vi "Lock Subpanel.vi"(8 "error in (no error)":errorcluster, 11 "Subpanel in":refnum<class "Subpanel.lvclass">) -> (0 "error out":errorcluster, 2 "semaphore":T1)   [LabVIEW 2017, in "MGI-Panel Manager.lvlib" / "Subpanel.lvclass"]
uses:
  Subpanel.lvclass
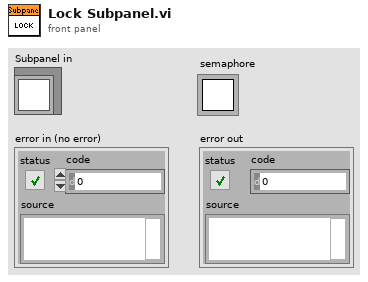
[diagram p1: front panel]
types:
  T1 = typedef "Semaphore RefNum" = refnum<k1>
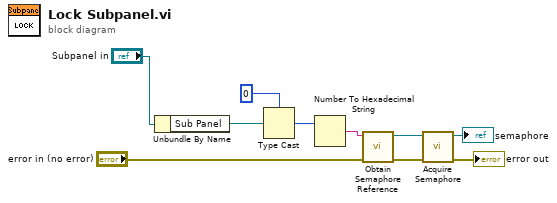
[diagram p0: block diagram]
diagram:
  n1 = Unbundle By Name("Subpanel in") -> ("Sub Panel"=w8:refnum<vi>)
  n2 = Type Cast(type=u32 0, x=w8) -> (*(type *) &x=w7:u32)
  n3 = Number To Hexadecimal String(2:w7) -> (0:w10:string)  [unwired: 1 in]
  n4 = call <vilib>:"Obtain Semaphore Reference.vi"("error in (no error)"="error in (no error)", "name (unnamed)"=w10) -> ("error out"=w3:errorcluster, "semaphore"=w4:T1)  [unwired: 3 in, 1 out]
  n5 = call <vilib>:"Acquire Semaphore.vi"("error in (no error)"=w3, "semaphore"=w4) -> ("error out"=→"error out":errorcluster, "semaphore out"=→"semaphore":T1)  [unwired: 3 in, 1 out]
